vi "STARLYTE.vi"() -> ()   [LabVIEW 2013]
doc: "# STARLYTE AI ENERGY SYSTEM\n# SUBMITTED FOR 2017 NASA INTERNATIONAL SPACE APPS CHALLENGE\n# PROJECT: STARLYTE\n# AUTHORS: ANDREW DENIO, KEVIN JOHNSON\n# DATE: 5/5/2017\n\n\nThis VI demonstrates how to use .Net Speech Recognition to control an application by Voice"
panel:
  out "Battery Storage (%)":dbl(slide) scale=0.0..100.0
  out "TIME":string
  out "Previous 7 Days":T1
  out "12 Day Forecast":T2
  out "Temperature (F)":dbl
  out "Sky Efficiency (%)":dbl
  out "Clearsky GHI (W/m2)":dbl
  in  "offsetHour":i32=-5
  in  "stop":bool
  out "current time":string
  out "current Temperature (deg C)":dbl format="%#_8g"
  out "Solar Radiation-GHI (W/m2)":dbl
  out "Instantaneous Power from the Solar Array":dbl
  out "Dew Point (c)":dbl format="%#_9g"
  out "Pressure (mbar)":dbl format="%#_7g"
  out "Relative Humidity (%)":dbl format="%#_8g"
  out "Precipitable Water (mm)":dbl format="%#_8g"
  out "Wind Direction (degree)":dbl format="%#_7g"
  out "Wind Speed (m/s)":dbl format="%#_9g"
  out "Solar Zenith Angle (degree)":dbl format="%#_7g"
  out "error out 2":errorcluster
  in  "Error in":errorcluster
  out "error out":errorcluster
  out "SpeechLib.ISpeechVoice 2":refnum<k7>
  in  "SpeechLib.ISpeechVoice":refnum<k7>
  out "Score":dbl
  in  "Phrases":i32(listbox)
  in  "Exit":bool
  out "Command":string
  # "HI-SEAS Artificial Intelligence Energy System"
  # "Start Microsoft Speech Engine \nBefore Running this App"
  # "Data for simulation provided by:"
  # "Daily Past Data       -7               -6              -5              -4              -3               -2              -1"
  # "Daily Future Data +1               +2              +3             +4             +5              +6              +7              +8             +9           +10            +11           +12"
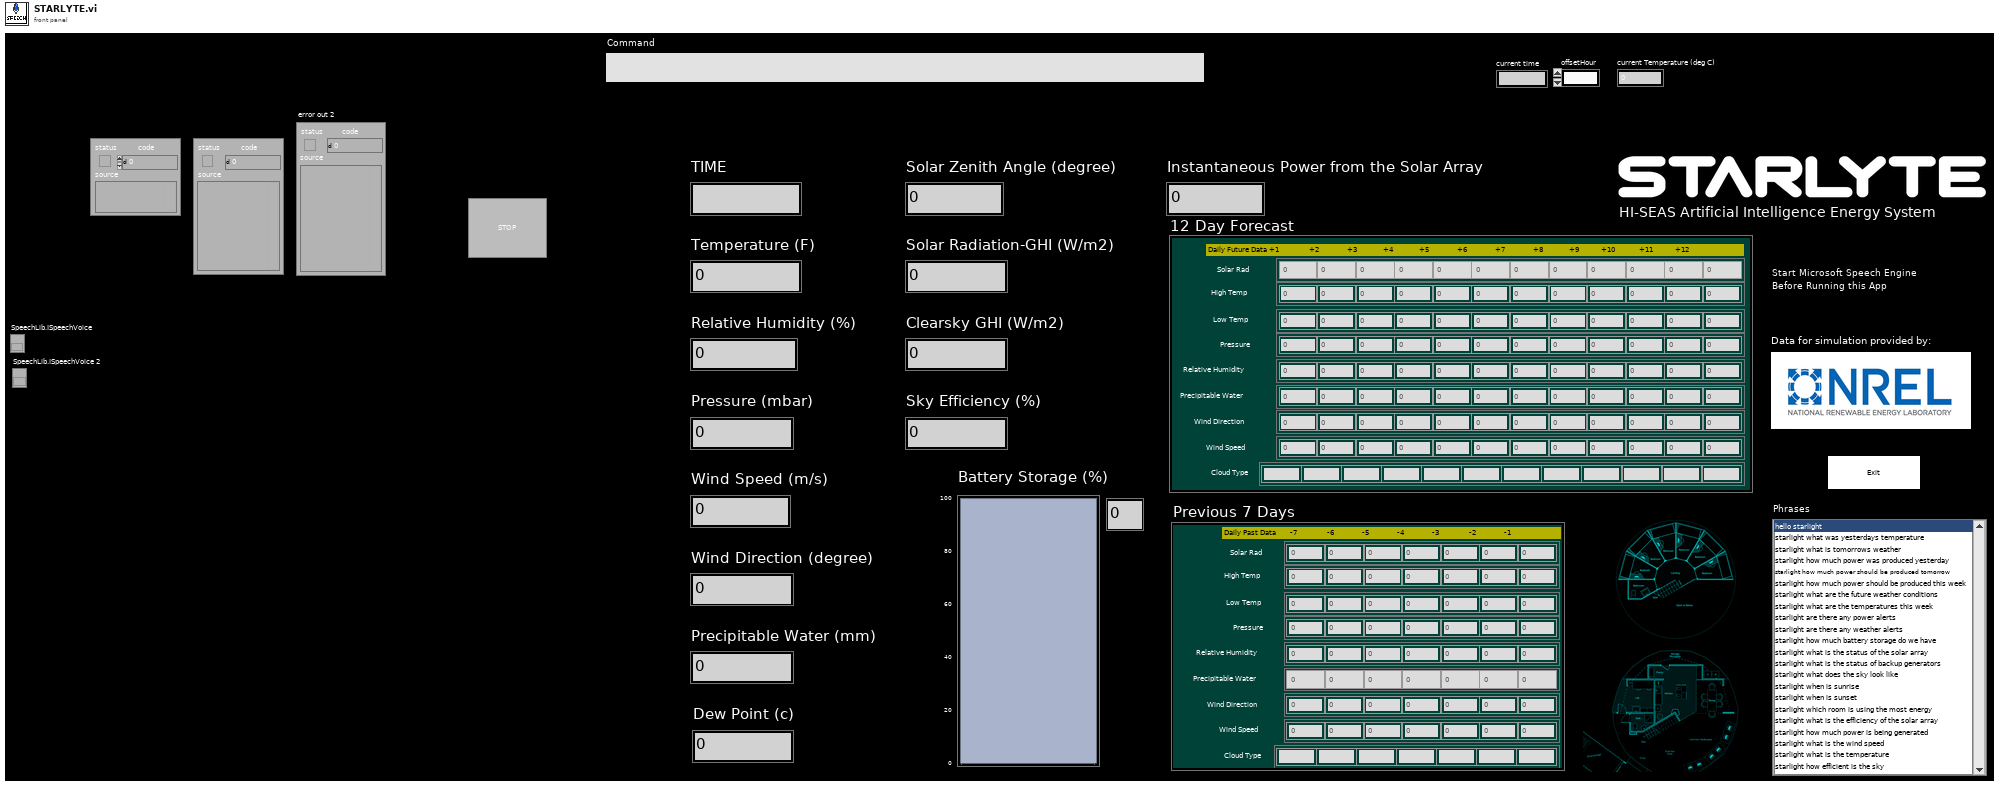
[diagram p1: front panel]
types:
  T1 = cluster{"Wind Speed":dbl[], "Wind Direction":dbl[], "Precipitable Water":dbl[], "Relative Humidity":dbl[], "Pressure":dbl[], "Low Temp":dbl[], "High Temp":dbl[], "Solar Rad":dbl[], "Cloud Type":string[]}
  T2 = cluster{"Solar Rad":dbl[], "High Temp":dbl[], "Low Temp":dbl[], "Pressure":dbl[], "Relative Humidity":dbl[], "Precipitable Water":dbl[], "Wind Direction":dbl[], "Wind Speed":dbl[], "Cloud Type":string[]}
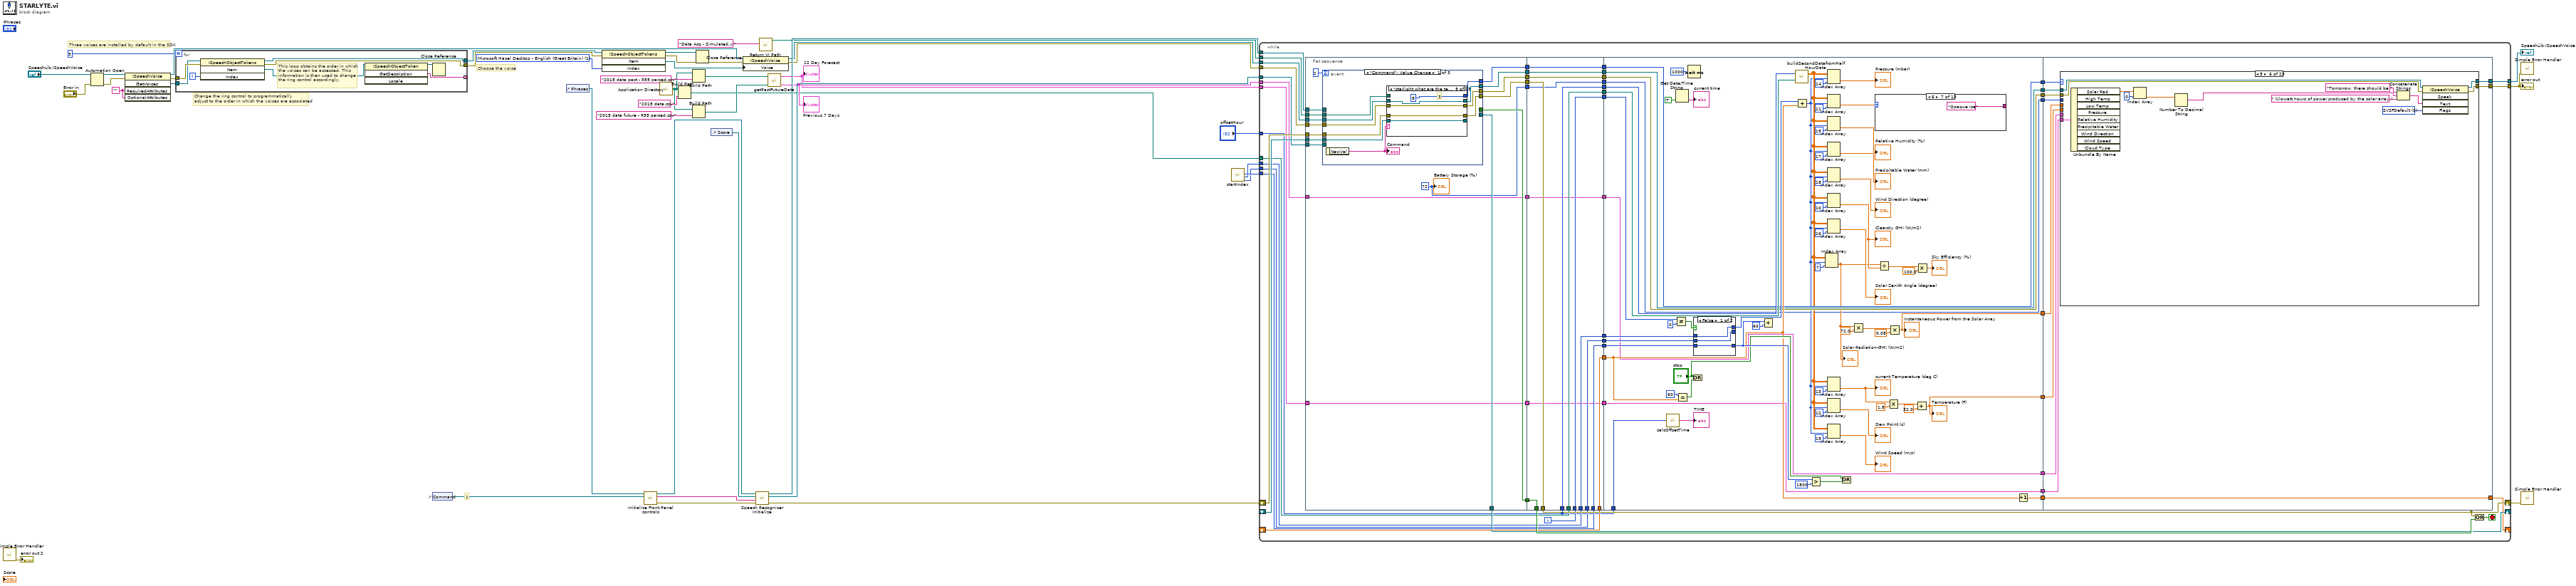
[diagram p0: block diagram]
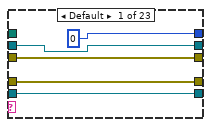
[diagram p2: hidden frame]
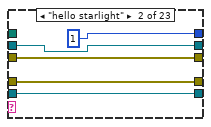
[diagram p3: hidden frame]
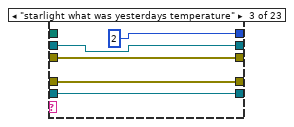
[diagram p4: hidden frame]
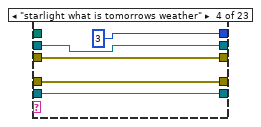
[diagram p5: hidden frame]
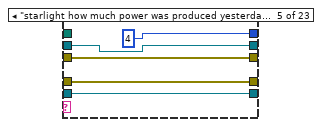
[diagram p6: hidden frame]
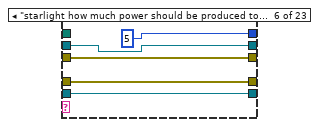
[diagram p7: hidden frame]
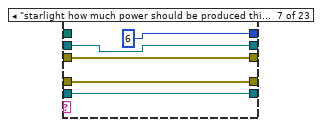
[diagram p8: hidden frame]
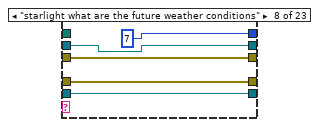
[diagram p9: hidden frame]
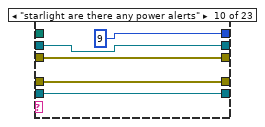
[diagram p10: hidden frame]
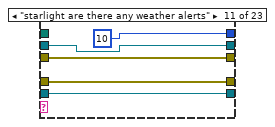
[diagram p11: hidden frame]
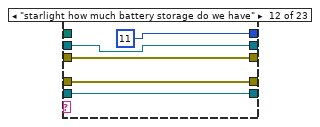
[diagram p12: hidden frame]
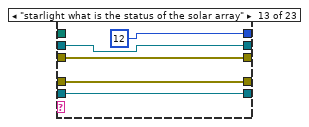
[diagram p13: hidden frame]
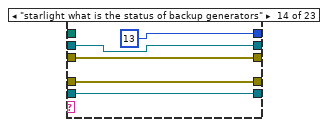
[diagram p14: hidden frame]
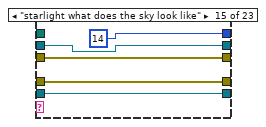
[diagram p15: hidden frame]
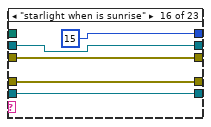
[diagram p16: hidden frame]
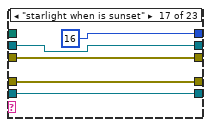
[diagram p17: hidden frame]
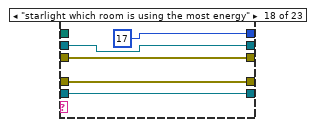
[diagram p18: hidden frame]
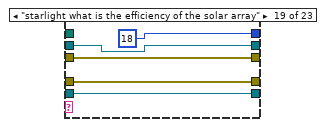
[diagram p19: hidden frame]
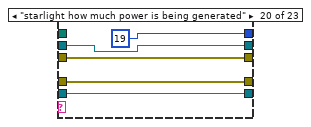
[diagram p20: hidden frame]
diagram:
  w31 = 1 items=["Microsoft David Desktop - English (United States)", "Microsoft Hazel Desktop - English (Great Britain)", "Microsoft Zira Desktop - English (United States)"] ("Choose the voice")
  w29 = ""
  # "Choose the voice"
  # "Three voices are installed by default in the SDK"
  # "Change the ring control to programmatically \nadjust to the order in which the voices are associated"
  # "1"
  n1 = call <vilib>:"Simple Error Handler.vi"() -> ("error out"=→"error out 2":errorcluster)  [unwired: 3 in, 6 out]
  n2 = Automation Open(error in (no error)="Error in", Automation Refnum="SpeechLib.ISpeechVoice") -> (Automation Refnum=w33:refnum<k7>, error out=w28:errorcluster)  [unwired: 2 in]
  n3 = invoke class="ISpeechVoice" method="GetVoices"(reference=w33, error in=w28, "RequiredAttributes"=w29, "OptionalAttributes"=w29) -> (reference out=w32:refnum<k7>, error out=w27:errorcluster, "GetVoices"=w26:refnum<k7>)  [unwired: 1 in, 2 out]
  n4 = for {
    N: 3 -> [_]
    tunnel: [w53] -> w21
    tunnel: w27 -> [w50]
    tunnel: w26 -> [w49]
    tunnel: [w48] -> w24
    tunnel: [w47] -> _ mode=indexing
    i -> [w52]
    # "This loop obtains the order in which\nthe voices can be accessed. This \ninformation is then used to change\nthe ring control accordingly."
    n5 = invoke class="ISpeechObjectTokens" method="Item"(reference=w49, error in=w50, "Index"=w52) -> (reference out=w48:refnum<k7>, error out=w53:errorcluster, "Item"=w54:refnum<k7>)  [unwired: 1 in, 1 out]
    n6 = invoke class="ISpeechObjectToken" method="GetDescription"(reference=w54) -> (reference out=w51:refnum<k7>, "GetDescription"=w47:string)  [unwired: 3 in, 2 out]
    n7 = Close Reference(reference=w51) -> ()  [unwired: 1 in, 1 out]
  }
  n8 = control-ref of="Command"() -> (w40:refnum<vi>)
  n9 = control-ref of="Phrases"() -> (w37:refnum<vi>)
  n10 = invoke class="ISpeechObjectTokens" method="Item"(reference=w24, error in=w21, "Index"=w31) -> (reference out=w23:refnum<k7>, error out=w20:errorcluster, "Item"=w30:refnum<k7>)  [unwired: 1 in, 1 out]
  n11 = call "Initialize Front Panel controls.vi"("Command"=w40, "ListBox in"=w37) -> ("error out"=w38:errorcluster, "Item Names"=w43:string[], "String out"=w41:refnum<vi>)  [unwired: 7 in]
  n12 = call <vilib>:"Application Directory.vi"() -> ("Application Directory"=w4:path)
  n13 = Build Path(base path=w4, name or relative path="2015 data.csv") -> (appended path=w1:path)
  n14 = Build Path(base path=w4, name or relative path="2015 data past - R55 parsed.csv") -> (appended path=w6:path)
  n15 = Build Path(base path=w4, name or relative path="2015 data future - R55 parsed.csv") -> (appended path=w5:path)
  n16 = Close Reference(reference=w23, error in (no error)=w20) -> (error out=w19:errorcluster)
  n17 = control-ref of="Score"() -> (w39:refnum<vi>)
  n18 = property class="ISpeechVoice"(reference=w32, error in=w19, "Voice"=w30) -> (reference out=w18:refnum<k7>, error out=w17:errorcluster)
  n19 = call "Speech Recognizer Initialize.vi"("Error In"=w38, "String[] phrases"=w43, "Score"=w39, "Text"=w41) -> ("error out"=w46:errorcluster, "Event Callback"=w45:refnum<k27>, "reference"=w44:refnum<k24>)  [unwired: 5 out]
  n20 = call "Return VI Path.vi"("name or relative path"="Data Acq - Simulated.vi") -> ("appended path"=w42:path)  [unwired: 10 in]
  n21 = call "getPastFutureData.vi"("2015 data future - R55 parsed.csv"=w5, "2015 data past - R55 parsed.csv"=w6) -> ("Data Past Cluster"=w3:T1, "Data Future Cluster"=w2:T2)  [unwired: 2 in]
  "12 Day Forecast" <- w2
  "Previous 7 Days" <- w3
  n22 = call "startIndex.vi"() -> ("Second"=w10:i32, "startIndex"=w11:i32, "minuteTOsecondStartIndex"=w12:i32)  [unwired: 4 in, 1 out]
  n23 = while {
    shift-right: [w99] -> w35
    shift-left: w46 -> [w107]
    tunnel: w45 -> [w105]
    tunnel: w44 -> [w104]
    tunnel: w42 -> [w103]
    shift-right: [w102] -> _
    shift-left: _ -> [w101]
    tunnel: w18 -> [w98]
    tunnel: w17 -> [w97]
    tunnel: [w72] -> w16
    tunnel: [w73] -> w15
    tunnel: "offsetHour" -> [w60]
    tunnel: w1 -> [w91]
    tunnel: w12 -> [w88]
    tunnel: w11 -> [w86]
    tunnel: w10 -> [w84]
    shift-right: [w81] -> _
    shift-left: _ -> [w79]
    tunnel: w3 -> [w68]
    tunnel: w2 -> [w61]
    i -> [w82]
    stop <- w100 stop-if-true
    n24 = flat-sequence {
      tunnel: w107 -> [w124]
      tunnel: w105 -> [w122]
      tunnel: w104 -> [w121]
      tunnel: w103 -> [w120]
      tunnel: [w113] -> w102
      tunnel: w101 -> [w119]
      tunnel: w98 -> [w117]
      tunnel: w97 -> [w116]
      tunnel: [w123] -> w96
      tunnel: [w118] -> w95
      tunnel: [w115] -> w94
      tunnel: [w114] -> w93
      tunnel: [w111] -> w69
      tunnel: w68 -> [w110]
      tunnel: [w110] -> w67
      tunnel: [w109] -> w62
      tunnel: w61 -> [w109]
      tunnel: [w108] -> w57
      tunnel: [w268] -> w99
      tunnel: [w269] -> w106
      tunnel: w96 -> [w269]
      tunnel: w95 -> [w268]
      tunnel: w94 -> [w259]
      tunnel: w93 -> [w260]
      tunnel: [w267] -> w92
      tunnel: w60 -> [w267]
      tunnel: w91 -> [w266]
      tunnel: [w266] -> w90
      tunnel: [w265] -> w89
      tunnel: w88 -> [w265]
      tunnel: [w264] -> w87
      tunnel: w86 -> [w264]
      tunnel: [w263] -> w85
      tunnel: w84 -> [w263]
      tunnel: [w262] -> w83
      tunnel: w82 -> [w262]
      tunnel: [w261] -> w80
      tunnel: w79 -> [w261]
      tunnel: [w260] -> w76
      tunnel: [w259] -> w74
      tunnel: [w258] -> w70
      tunnel: w69 -> [w258]
      tunnel: w67 -> [w257]
      tunnel: [w257] -> w65
      tunnel: [w256] -> w63
      tunnel: w62 -> [w256]
      tunnel: [w255] -> w58
      tunnel: w57 -> [w255]
      tunnel: w92 -> [w329]
      tunnel: w90 -> [w328]
      tunnel: w89 -> [w327]
      tunnel: w87 -> [w326]
      tunnel: w85 -> [w325]
      tunnel: w83 -> [w324]
      tunnel: w80 -> [w295]
      tunnel: [w319] -> w78
      tunnel: [w294] -> w77
      tunnel: w76 -> [w294]
      tunnel: [w293] -> w75
      tunnel: w74 -> [w293]
      tunnel: [w291] -> w71
      tunnel: w70 -> [w291]
      tunnel: [w276] -> w66
      tunnel: w65 -> [w276]
      tunnel: [w275] -> w64
      tunnel: w63 -> [w275]
      tunnel: w60 -> [w273]
      tunnel: [w272] -> w59
      tunnel: w58 -> [w272]
      tunnel: [w271] -> w56
      tunnel: [w270] -> w55
      tunnel: [w361] -> w81
      tunnel: w78 -> [w361]
      tunnel: w77 -> [w360]
      tunnel: w75 -> [w359]
      tunnel: [w358] -> w73
      tunnel: [w357] -> w72
      tunnel: w71 -> [w356]
      tunnel: w66 -> [w355]
      tunnel: w64 -> [w354]
      tunnel: w59 -> [w353]
      tunnel: w56 -> [w352]
      tunnel: w55 -> [w351]
      frame #0 {
        w108 = 72
        n25 = event shown="[0] \"Command\": Value Change" {
          selector: _ -> [_ _ _]
          dyn-events: _ -> [_ _ _]
          timeout: 2 -> [_ _ _]
          tunnel: w124 -> [w134 _ w251]
          tunnel: [_ _ "Exit"] -> w123
          tunnel: [w133 _ w251] -> w118
          tunnel: w122 -> [_ _ w253]
          tunnel: w121 -> [_ _ w252]
          tunnel: w120 -> [w131 _ _]
          tunnel: w119 -> [w130 _ _]
          tunnel: w117 -> [w129 _ _]
          tunnel: w116 -> [w128 _ _]
          tunnel: [w127 _ _] -> w115
          tunnel: [w126 _ _] -> w114
          tunnel: [_ _ refnum<vi> refnum ("vi reference")] -> w113
          tunnel: [w125 _ _] -> w111
          event "Command": Value Change {
            # "3"
            n26 = event-data() -> ("NewVal"=w132:string)  [unwired: 1 out]
            "Command" <- w132
            n27 = case shown="\"starlight what are the temperatures this week\"" w132 {
              tunnel: w134 -> [w139 w144 w149 w154 w159 w164 w169 w174 w179 w184 w189 w194 w199 w204 w209 w214 w219 w224 w229 w234 w239 w244 w249]
              tunnel: [w139 w144 w149 w154 w159 w164 w169 w174 w179 w184 w189 w194 w199 w204 w209 w214 w219 w224 w229 w234 w239 w244 w249] -> w133
              tunnel: w131 -> [_ _ _ _ _ _ _ _ _ _ _ _ _ _ _ _ _ _ _ _ _ _ _]
              tunnel: [w138 w143 w148 w153 w158 w163 w168 w173 w178 w183 w188 w193 w198 w203 w208 w213 w218 w223 w228 w233 w238 w243 w248] -> _
              tunnel: w130 -> [w138 w143 w148 w153 w158 w163 w168 w173 w178 w183 w188 w193 w198 w203 w208 w213 w218 w223 w228 w233 w238 w243 w248]
              tunnel: w129 -> [w137 w142 w147 w152 w157 w162 w167 w172 w177 w182 w187 w192 w197 w202 w207 w212 w217 w222 w227 w232 w237 w242 w247]
              tunnel: w128 -> [w136 w141 w146 w151 w156 w161 w166 w171 w176 w181 w186 w191 w196 w201 w206 w211 w216 w221 w226 w231 w236 w241 w246]
              tunnel: [w136 w141 w146 w151 w156 w161 w166 w171 w176 w181 w186 w191 w196 w201 w206 w211 w216 w221 w226 w231 w236 w241 w246] -> w127
              tunnel: [w137 w142 w147 w152 w157 w162 w167 w172 w177 w182 w187 w192 w197 w202 w207 w212 w217 w222 w227 w232 w237 w242 w247] -> w126
              tunnel: [0 1 2 3 4 5 6 7 8 9 10 11 12 13 14 15 16 17 18 19 20 21 22] -> w125
              frame Default {
              }
              frame "hello starlight" {
              }
              frame "starlight what was yesterdays temperature" {
              }
              frame "starlight what is tomorrows weather" {
              }
              frame "starlight how much power was produced yesterday" {
              }
              frame "starlight how much power should be produced tomorrow" {
              }
              frame "starlight how much power should be produced this week" {
              }
              frame "starlight what are the future weather conditions" {
              }
              frame "starlight what are the temperatures this week" {
              }
              frame "starlight are there any power alerts" {
              }
              frame "starlight are there any weather alerts" {
              }
              frame "starlight how much battery storage do we have" {
              }
              frame "starlight what is the status of the solar array" {
              }
              frame "starlight what is the status of backup generators" {
              }
              frame "starlight what does the sky look like" {
              }
              frame "starlight when is sunrise" {
              }
              frame "starlight when is sunset" {
              }
              frame "starlight which room is using the most energy" {
              }
              frame "starlight what is the efficiency of the solar array" {
              }
              frame "starlight how much power is being generated" {
              }
              frame "starlight what is the wind speed" {
              }
              frame "starlight what is the temperature" {
              }
              frame "starlight how efficient is the sky" {
              }
            }
          }
          event Timeout {
            n28 = event-data() -> ()  [unwired: 2 out]
          }
          event "Exit": Value Change {
            # "4"
            n29 = event-data() -> ()  [unwired: 2 out]
            n30 = Unregister For Events(event registration refnum=w253) -> ()  [unwired: 1 in, 1 out]
            n31 = Close Reference(reference=w252) -> ()  [unwired: 1 in, 1 out]
          }
        }
        "Battery Storage (%)" <- w108
      }
      frame #1 {
      }
      frame #2 {
        n32 = call "calcOffsetTime.vi"("Hour Offset"=w273) -> ("currentTimeOffset"=→"TIME":string)  [unwired: 4 in]
        n33 = Not Equal?(x=w324, y=0) -> (x != y?=w331:bool)
        n34 = Get Date/Time String(want seconds? (F)=TRUE) -> (time string=→"current time":string)  [unwired: 2 in, 1 out]
        n35 = Equal?(x=60, y=w295) -> (x = y?=w314:bool)
        n36 = Wait (ms)(milliseconds to wait=u32 1000) -> ()  [unwired: 1 out]
        n37 = Or(x="stop", y=w314) -> ()  [unwired: 1 out]
        n38 = case shown="False" w331 {
          tunnel: w325 -> [w349 _]
          tunnel: [w349 w350] -> _
          tunnel: w327 -> [w348 _]
          tunnel: [w348 w350] -> w332
          tunnel: [w347 w350] -> w333
          tunnel: w326 -> [w347 _]
          frame False {
          }
          frame True {
            w350 = 0 ("x")
          }
        }
        n39 = Add(x=w332, y=60 ("x")) -> ()  [unwired: 1 out]
        n40 = call "buildSecondDatafromHalfHourData.vi"("2015 data.csv"=w328, "offsetHour"=w329) -> ("Array"=w284:dbl[][])  [unwired: 1 in]
        n41 = Add(x=w333, y=w295) -> (x+y=w283:i32)
        n42 = Greater?(x=w332, y=1800 ("x")) -> (0:w323:bool)
        n43 = Index Array(array=w284, index (row)=w283, index (col)=7 ("disabled index (col)")) -> (element=w288:dbl)
        "Solar Radiation-GHI (W/m2)" <- w288
        n44 = Index Array(array=w284, index (row)=w283, index (col)=14 ("disabled index (col)")) -> (element=→"Pressure (mbar)":dbl)
        n45 = Index Array(array=w284, index (row)=w283, index (col)=11 ("disabled index (col)")) -> (element=w281:dbl)
        n46 = Index Array(array=w284, index (row)=w283, index (col)=15 ("disabled index (col)")) -> (element=→"Relative Humidity (%)":dbl)
        n47 = Index Array(array=w284, index (row)=w283, index (col)=17 ("disabled index (col)")) -> (element=→"Precipitable Water (mm)":dbl)
        n48 = Index Array(array=w284, index (row)=w283, index (col)=18 ("disabled index (col)")) -> (element=→"Wind Direction (degree)":dbl)
        n49 = Index Array(array=w284, index (row)=w283, index (col)=10 ("disabled index (col)")) -> (element=w289:dbl)
        "Clearsky GHI (W/m2)" <- w289
        n50 = Index Array(array=w284, index (row)=w283, index (col)=16 ("disabled index (col)")) -> (element=→"Solar Zenith Angle (degree)":dbl)
        n51 = Index Array(array=w284, index (row)=w283, index (col)=13 ("disabled index (col)")) -> (element=w278:dbl)
        "current Temperature (deg C)" <- w278
        n52 = Index Array(array=w284, index (row)=w283, index (col)=12 ("disabled index (col)")) -> (element=→"Dew Point (c)":dbl)
        n53 = Index Array(array=w284, index (row)=w283, index (col)=19 ("disabled index (col)")) -> (element=→"Wind Speed (m/s)":dbl)
        n54 = Or(x="stop", y=w323) -> ()  [unwired: 1 out]
        n55 = Multiply(x=w288, y=72.0) -> (x*y=w303:dbl)
        n56 = case shown="6" w281 {
          tunnel: ["Clear" "Probably Clear" "Fog" "Water" "Super-Cooled Water" "Mixed" "Opaque Ice" "Cirrus" "Overlapping" "Overshooting" "Unknown" "Dust" "Smoke"] -> _
          frame 0 {
          }
          frame 1 {
          }
          frame 2 {
          }
          frame 3 {
          }
          frame 4 {
          }
          frame 5 {
          }
          frame 6 {
          }
          frame 7 {
          }
          frame 8 {
          }
          frame 9 {
          }
          frame 10, Default {
          }
          frame 11 {
          }
          frame 12 {
          }
        }
        n57 = Divide(x=w288, y=w289) -> (x/y=w287:dbl)
        n58 = Multiply(x=w278, y=1.8) -> (x*y=w280:dbl)
        n59 = Multiply(x=w303, y=0.08) -> (x*y=w271:dbl)
        "Instantaneous Power from the Solar Array" <- w271
        n60 = Add(x=w280, y=32.0) -> (x+y=w270:dbl)
        "Temperature (F)" <- w270
        n61 = Multiply(x=w287, y=100.0) -> (x*y=→"Sky Efficiency (%)":dbl)
        n62 = Increment(x=w295) -> (x+1=w319:dbl)
      }
      frame #3 {
        n63 = case shown="5" w356 {
          tunnel: w360 -> [w362 w368 w394 w442 w455 w468 w474 w480 w486 w492 w498 w508 w514 w520 w526 w532 w538 w544 w550 w560 w566 w576 w582]
          tunnel: w359 -> [w363 w367 w393 w441 w454 w467 w473 w479 w485 w491 w497 w507 w513 w519 w525 w531 w537 w543 w549 w559 w565 w575 w581]
          tunnel: [w362 w366 w392 w440 w453 w466 w472 w478 w484 w490 w496 w506 w512 w518 w524 w530 w536 w542 w548 w558 w564 w574 w580] -> w358
          tunnel: [w363 w365 w391 w439 w452 w465 w471 w477 w483 w489 w495 w505 w511 w517 w523 w529 w535 w541 w547 w557 w563 w573 w579] -> w357
          tunnel: w355 -> [_ _ w390 _ w451 _ _ _ _ _ _ _ _ _ _ _ _ _ _ _ _ _ _]
          tunnel: w354 -> [_ _ _ w438 _ w464 _ _ _ _ _ _ _ _ _ _ _ _ _ _ _ _ _]
          tunnel: w353 -> [_ _ _ _ _ _ _ _ _ _ _ w503 _ _ _ _ _ _ _ _ _ _ _]
          tunnel: w352 -> [_ _ _ _ _ _ _ _ _ _ _ _ _ _ _ _ _ _ _ w556 _ _ _]
          tunnel: w351 -> [_ _ _ _ _ _ _ _ _ _ _ _ _ _ _ _ _ _ _ _ _ w569 _]
          frame 0, Default {
          }
          frame 1 {
            w369 = 0 items=["SVSFDefault"=0, "SVSFlagsAsync"=1, "SVSFPurgeBeforeSpeak"=2, "SVSFIsFilename"=4, "SVSFIsXML"=8, "SVSFIsNotXML"=16, "SVSFPersistXML"=32, "SVSFNLPSpeakPunc, SVSFNLPMask"=64, "SVSFVoiceMask"=127, "SVSFUnusedFlags"=-128] ("Flags")
            n64 = invoke class="ISpeechVoice" method="Speak"(reference=w368, error in=w367, "Text"="Hello crew mate Denio", "Flags"=w369) -> (reference out=w366:refnum<k7>, error out=w365:errorcluster)  [unwired: 1 in, 3 out]
          }
          frame 2 {
            w395 = 0 items=["SVSFDefault"=0, "SVSFlagsAsync"=1, "SVSFPurgeBeforeSpeak"=2, "SVSFIsFilename"=4, "SVSFIsXML"=8, "SVSFIsNotXML"=16, "SVSFPersistXML"=32, "SVSFNLPSpeakPunc, SVSFNLPMask"=64, "SVSFVoiceMask"=127, "SVSFUnusedFlags"=-128] ("Flags")
            n65 = Unbundle By Name(w390) -> ("Low Temp"=w389:dbl[], "High Temp"=w386:dbl[])  [unwired: 7 out]
            n66 = Index Array(array=w386, index=6) -> (element=w375:dbl)
            n67 = Index Array(array=w389, index=6) -> (element=w381:dbl)
            n68 = Multiply(x=w375, y=1.8) -> (x*y=w378:dbl)
            n69 = Multiply(x=w381, y=1.8) -> (x*y=w382:dbl)
            n70 = Add(x=w378, y=32.0) -> (x+y=w379:dbl)
            n71 = Add(x=w382, y=32.0) -> (x+y=w380:dbl)
            n72 = Number To Decimal String(number=w379) -> (decimal integer string=w374:string)  [unwired: 1 in]
            n73 = Number To Decimal String(number=w380) -> (decimal integer string=w372:string)  [unwired: 1 in]
            n74 = Concatenate Strings("Yesterday, the high temperature was " ("string"), w374, " degrees farenheit and the low temperature was " ("string"), w372, " degrees farenheit" ("string")) -> (w370:string)
            n75 = invoke class="ISpeechVoice" method="Speak"(reference=w394, error in=w393, "Text"=w370, "Flags"=w395) -> (reference out=w392:refnum<k7>, error out=w391:errorcluster)  [unwired: 1 in, 3 out]
          }
          frame 3 {
            w443 = 0 items=["SVSFDefault"=0, "SVSFlagsAsync"=1, "SVSFPurgeBeforeSpeak"=2, "SVSFIsFilename"=4, "SVSFIsXML"=8, "SVSFIsNotXML"=16, "SVSFPersistXML"=32, "SVSFNLPSpeakPunc, SVSFNLPMask"=64, "SVSFVoiceMask"=127, "SVSFUnusedFlags"=-128] ("Flags")
            n76 = Unbundle By Name(w438) -> ("Solar Rad"=w423:dbl[], "High Temp"=w431:dbl[], "Low Temp"=w424:dbl[], "Pressure"=w418:dbl[], "Relative Humidity"=w414:dbl[], "Precipitable Water"=w410:dbl[], "Wind Direction"=w406:dbl[], "Wind Speed"=w413:dbl[])  [unwired: 1 out]
            n77 = Index Array(array=w431, index=0) -> (element=w436:dbl)
            n78 = Index Array(array=w424, index=0) -> (element=w426:dbl)
            n79 = Index Array(array=w423, index=0) -> (element=w421:dbl)
            n80 = Index Array(array=w418, index=0) -> (element=w419:dbl)
            n81 = Index Array(array=w414, index=0) -> (element=w412:dbl)
            n82 = Index Array(array=w410, index=0) -> (element=w409:dbl)
            n83 = Index Array(array=w406, index=0) -> (element=w408:dbl)
            n84 = Index Array(array=w413, index=0) -> (element=w411:dbl)
            n85 = Number To Decimal String(number=w421) -> ()  [unwired: 1 in, 1 out]
            n86 = Number To Decimal String(number=w419) -> ()  [unwired: 1 in, 1 out]
            n87 = Number To Decimal String(number=w409) -> ()  [unwired: 1 in, 1 out]
            n88 = Number To Decimal String(number=w408) -> ()  [unwired: 1 in, 1 out]
            n89 = Number To Decimal String(number=w412) -> (decimal integer string=w399:string)  [unwired: 1 in]
            n90 = Number To Decimal String(number=w411) -> (decimal integer string=w396:string)  [unwired: 1 in]
            n91 = Multiply(x=w436, y=1.8) -> (x*y=w435:dbl)
            n92 = Multiply(x=w426, y=1.8) -> (x*y=w427:dbl)
            n93 = Add(x=w435, y=32.0) -> (x+y=w437:dbl)
            n94 = Add(x=w427, y=32.0) -> (x+y=w425:dbl)
            n95 = Number To Decimal String(number=w437) -> (decimal integer string=w404:string)  [unwired: 1 in]
            n96 = Number To Decimal String(number=w425) -> (decimal integer string=w401:string)  [unwired: 1 in]
            n97 = Concatenate Strings("Tomrrow, the high temperature will be " ("string"), w404, " degrees farenheit, and the low temperature will be " ("string"), w401, " degrees farenheit, The humidity will be " ("string"), w399, " percent, and the wind speed will reach " ("string"), w396, " miles per hour." ("string")) -> (w402:string)
            n98 = invoke class="ISpeechVoice" method="Speak"(reference=w442, error in=w441, "Text"=w402, "Flags"=w443) -> (reference out=w440:refnum<k7>, error out=w439:errorcluster)  [unwired: 1 in, 3 out]
          }
          frame 4 {
            w456 = 0 items=["SVSFDefault"=0, "SVSFlagsAsync"=1, "SVSFPurgeBeforeSpeak"=2, "SVSFIsFilename"=4, "SVSFIsXML"=8, "SVSFIsNotXML"=16, "SVSFPersistXML"=32, "SVSFNLPSpeakPunc, SVSFNLPMask"=64, "SVSFVoiceMask"=127, "SVSFUnusedFlags"=-128] ("Flags")
            n99 = Unbundle By Name(w451) -> ("Solar Rad"=w448:dbl[])  [unwired: 8 out]
            n100 = Index Array(array=w448, index=0) -> (element=w450:dbl)
            n101 = Number To Decimal String(number=w450) -> (decimal integer string=w446:string)  [unwired: 1 in]
            n102 = Concatenate Strings("Yesterday, there were " ("string"), w446, " kilowatt hours produced from the solar array." ("string")) -> (w444:string)
            n103 = invoke class="ISpeechVoice" method="Speak"(reference=w455, error in=w454, "Text"=w444, "Flags"=w456) -> (reference out=w453:refnum<k7>, error out=w452:errorcluster)  [unwired: 1 in, 3 out]
          }
          frame 5 {
            w469 = 0 items=["SVSFDefault"=0, "SVSFlagsAsync"=1, "SVSFPurgeBeforeSpeak"=2, "SVSFIsFilename"=4, "SVSFIsXML"=8, "SVSFIsNotXML"=16, "SVSFPersistXML"=32, "SVSFNLPSpeakPunc, SVSFNLPMask"=64, "SVSFVoiceMask"=127, "SVSFUnusedFlags"=-128] ("Flags")
            n104 = Unbundle By Name(w464) -> ("Solar Rad"=w463:dbl[])  [unwired: 8 out]
            n105 = Index Array(array=w463, index=0) -> (element=w461:dbl)
            n106 = Number To Decimal String(number=w461) -> (decimal integer string=w458:string)  [unwired: 1 in]
            n107 = Concatenate Strings("Tomorrow, there should be " ("string"), w458, " kilowatt hours of power produced by the solar array." ("string")) -> (w460:string)
            n108 = invoke class="ISpeechVoice" method="Speak"(reference=w468, error in=w467, "Text"=w460, "Flags"=w469) -> (reference out=w466:refnum<k7>, error out=w465:errorcluster)  [unwired: 1 in, 3 out]
          }
          frame 6 {
            w475 = 0 items=["SVSFDefault"=0, "SVSFlagsAsync"=1, "SVSFPurgeBeforeSpeak"=2, "SVSFIsFilename"=4, "SVSFIsXML"=8, "SVSFIsNotXML"=16, "SVSFPersistXML"=32, "SVSFNLPSpeakPunc, SVSFNLPMask"=64, "SVSFVoiceMask"=127, "SVSFUnusedFlags"=-128] ("Flags")
            n109 = invoke class="ISpeechVoice" method="Speak"(reference=w474, error in=w473, "Text"=" ", "Flags"=w475) -> (reference out=w472:refnum<k7>, error out=w471:errorcluster)  [unwired: 1 in, 3 out]
          }
          frame 7 {
            w481 = 0 items=["SVSFDefault"=0, "SVSFlagsAsync"=1, "SVSFPurgeBeforeSpeak"=2, "SVSFIsFilename"=4, "SVSFIsXML"=8, "SVSFIsNotXML"=16, "SVSFPersistXML"=32, "SVSFNLPSpeakPunc, SVSFNLPMask"=64, "SVSFVoiceMask"=127, "SVSFUnusedFlags"=-128] ("Flags")
            n110 = invoke class="ISpeechVoice" method="Speak"(reference=w480, error in=w479, "Text"=" ", "Flags"=w481) -> (reference out=w478:refnum<k7>, error out=w477:errorcluster)  [unwired: 1 in, 3 out]
          }
          frame 8 {
            w487 = 0 items=["SVSFDefault"=0, "SVSFlagsAsync"=1, "SVSFPurgeBeforeSpeak"=2, "SVSFIsFilename"=4, "SVSFIsXML"=8, "SVSFIsNotXML"=16, "SVSFPersistXML"=32, "SVSFNLPSpeakPunc, SVSFNLPMask"=64, "SVSFVoiceMask"=127, "SVSFUnusedFlags"=-128] ("Flags")
            n111 = invoke class="ISpeechVoice" method="Speak"(reference=w486, error in=w485, "Text"=" ", "Flags"=w487) -> (reference out=w484:refnum<k7>, error out=w483:errorcluster)  [unwired: 1 in, 3 out]
          }
          frame 9 {
            w493 = 0 items=["SVSFDefault"=0, "SVSFlagsAsync"=1, "SVSFPurgeBeforeSpeak"=2, "SVSFIsFilename"=4, "SVSFIsXML"=8, "SVSFIsNotXML"=16, "SVSFPersistXML"=32, "SVSFNLPSpeakPunc, SVSFNLPMask"=64, "SVSFVoiceMask"=127, "SVSFUnusedFlags"=-128] ("Flags")
            n112 = invoke class="ISpeechVoice" method="Speak"(reference=w492, error in=w491, "Text"="There are no power alerts, Solar array performance is optimal ", "Flags"=w493) -> (reference out=w490:refnum<k7>, error out=w489:errorcluster)  [unwired: 1 in, 3 out]
          }
          frame 10 {
            w499 = 0 items=["SVSFDefault"=0, "SVSFlagsAsync"=1, "SVSFPurgeBeforeSpeak"=2, "SVSFIsFilename"=4, "SVSFIsXML"=8, "SVSFIsNotXML"=16, "SVSFPersistXML"=32, "SVSFNLPSpeakPunc, SVSFNLPMask"=64, "SVSFVoiceMask"=127, "SVSFUnusedFlags"=-128] ("Flags")
            n113 = invoke class="ISpeechVoice" method="Speak"(reference=w498, error in=w497, "Text"="There are no weather alerts at this time. ", "Flags"=w499) -> (reference out=w496:refnum<k7>, error out=w495:errorcluster)  [unwired: 1 in, 3 out]
          }
          frame 11 {
            w509 = 0 items=["SVSFDefault"=0, "SVSFlagsAsync"=1, "SVSFPurgeBeforeSpeak"=2, "SVSFIsFilename"=4, "SVSFIsXML"=8, "SVSFIsNotXML"=16, "SVSFPersistXML"=32, "SVSFNLPSpeakPunc, SVSFNLPMask"=64, "SVSFVoiceMask"=127, "SVSFUnusedFlags"=-128] ("Flags")
            n114 = Number To Decimal String(number=w503) -> (decimal integer string=w502:string)  [unwired: 1 in]
            n115 = Concatenate Strings("The battery storage is currently at " ("string"), w502, " percent" ("string")) -> (w500:string)
            n116 = invoke class="ISpeechVoice" method="Speak"(reference=w508, error in=w507, "Text"=w500, "Flags"=w509) -> (reference out=w506:refnum<k7>, error out=w505:errorcluster)  [unwired: 1 in, 3 out]
          }
          frame 12 {
            w515 = 0 items=["SVSFDefault"=0, "SVSFlagsAsync"=1, "SVSFPurgeBeforeSpeak"=2, "SVSFIsFilename"=4, "SVSFIsXML"=8, "SVSFIsNotXML"=16, "SVSFPersistXML"=32, "SVSFNLPSpeakPunc, SVSFNLPMask"=64, "SVSFVoiceMask"=127, "SVSFUnusedFlags"=-128] ("Flags")
            n117 = invoke class="ISpeechVoice" method="Speak"(reference=w514, error in=w513, "Text"="The solar array is functional, but panel number twenty five is below specifications ", "Flags"=w515) -> (reference out=w512:refnum<k7>, error out=w511:errorcluster)  [unwired: 1 in, 3 out]
          }
          frame 13 {
            w521 = 0 items=["SVSFDefault"=0, "SVSFlagsAsync"=1, "SVSFPurgeBeforeSpeak"=2, "SVSFIsFilename"=4, "SVSFIsXML"=8, "SVSFIsNotXML"=16, "SVSFPersistXML"=32, "SVSFNLPSpeakPunc, SVSFNLPMask"=64, "SVSFVoiceMask"=127, "SVSFUnusedFlags"=-128] ("Flags")
            n118 = invoke class="ISpeechVoice" method="Speak"(reference=w520, error in=w519, "Text"=" ", "Flags"=w521) -> (reference out=w518:refnum<k7>, error out=w517:errorcluster)  [unwired: 1 in, 3 out]
          }
          frame 14 {
            w527 = 0 items=["SVSFDefault"=0, "SVSFlagsAsync"=1, "SVSFPurgeBeforeSpeak"=2, "SVSFIsFilename"=4, "SVSFIsXML"=8, "SVSFIsNotXML"=16, "SVSFPersistXML"=32, "SVSFNLPSpeakPunc, SVSFNLPMask"=64, "SVSFVoiceMask"=127, "SVSFUnusedFlags"=-128] ("Flags")
            n119 = invoke class="ISpeechVoice" method="Speak"(reference=w526, error in=w525, "Text"=" ", "Flags"=w527) -> (reference out=w524:refnum<k7>, error out=w523:errorcluster)  [unwired: 1 in, 3 out]
          }
          frame 15 {
            w533 = 0 items=["SVSFDefault"=0, "SVSFlagsAsync"=1, "SVSFPurgeBeforeSpeak"=2, "SVSFIsFilename"=4, "SVSFIsXML"=8, "SVSFIsNotXML"=16, "SVSFPersistXML"=32, "SVSFNLPSpeakPunc, SVSFNLPMask"=64, "SVSFVoiceMask"=127, "SVSFUnusedFlags"=-128] ("Flags")
            n120 = invoke class="ISpeechVoice" method="Speak"(reference=w532, error in=w531, "Text"="Tomorrow, the sunrise will occur at five fifty two a m ", "Flags"=w533) -> (reference out=w530:refnum<k7>, error out=w529:errorcluster)  [unwired: 1 in, 3 out]
          }
          frame 16 {
            w539 = 0 items=["SVSFDefault"=0, "SVSFlagsAsync"=1, "SVSFPurgeBeforeSpeak"=2, "SVSFIsFilename"=4, "SVSFIsXML"=8, "SVSFIsNotXML"=16, "SVSFPersistXML"=32, "SVSFNLPSpeakPunc, SVSFNLPMask"=64, "SVSFVoiceMask"=127, "SVSFUnusedFlags"=-128] ("Flags")
            n121 = invoke class="ISpeechVoice" method="Speak"(reference=w538, error in=w537, "Text"="Tonight, sunset will occur at six forty three p m ", "Flags"=w539) -> (reference out=w536:refnum<k7>, error out=w535:errorcluster)  [unwired: 1 in, 3 out]
          }
          frame 17 {
            w545 = 0 items=["SVSFDefault"=0, "SVSFlagsAsync"=1, "SVSFPurgeBeforeSpeak"=2, "SVSFIsFilename"=4, "SVSFIsXML"=8, "SVSFIsNotXML"=16, "SVSFPersistXML"=32, "SVSFNLPSpeakPunc, SVSFNLPMask"=64, "SVSFVoiceMask"=127, "SVSFUnusedFlags"=-128] ("Flags")
            n122 = invoke class="ISpeechVoice" method="Speak"(reference=w544, error in=w543, "Text"="The current room using the most energy is the kitchen. ", "Flags"=w545) -> (reference out=w542:refnum<k7>, error out=w541:errorcluster)  [unwired: 1 in, 3 out]
          }
          frame 18 {
            w551 = 0 items=["SVSFDefault"=0, "SVSFlagsAsync"=1, "SVSFPurgeBeforeSpeak"=2, "SVSFIsFilename"=4, "SVSFIsXML"=8, "SVSFIsNotXML"=16, "SVSFPersistXML"=32, "SVSFNLPSpeakPunc, SVSFNLPMask"=64, "SVSFVoiceMask"=127, "SVSFUnusedFlags"=-128] ("Flags")
            n123 = invoke class="ISpeechVoice" method="Speak"(reference=w550, error in=w549, "Text"=" ", "Flags"=w551) -> (reference out=w548:refnum<k7>, error out=w547:errorcluster)  [unwired: 1 in, 3 out]
          }
          frame 19 {
            w561 = 0 items=["SVSFDefault"=0, "SVSFlagsAsync"=1, "SVSFPurgeBeforeSpeak"=2, "SVSFIsFilename"=4, "SVSFIsXML"=8, "SVSFIsNotXML"=16, "SVSFPersistXML"=32, "SVSFNLPSpeakPunc, SVSFNLPMask"=64, "SVSFVoiceMask"=127, "SVSFUnusedFlags"=-128] ("Flags")
            n124 = Number To Decimal String(number=w556) -> (decimal integer string=w554:string)  [unwired: 1 in]
            n125 = Concatenate Strings("Right now, there are " ("string"), w554, " watts being produced by the solar array" ("string")) -> (w552:string)
            n126 = invoke class="ISpeechVoice" method="Speak"(reference=w560, error in=w559, "Text"=w552, "Flags"=w561) -> (reference out=w558:refnum<k7>, error out=w557:errorcluster)  [unwired: 1 in, 3 out]
          }
          frame 20 {
            w567 = 0 items=["SVSFDefault"=0, "SVSFlagsAsync"=1, "SVSFPurgeBeforeSpeak"=2, "SVSFIsFilename"=4, "SVSFIsXML"=8, "SVSFIsNotXML"=16, "SVSFPersistXML"=32, "SVSFNLPSpeakPunc, SVSFNLPMask"=64, "SVSFVoiceMask"=127, "SVSFUnusedFlags"=-128] ("Flags")
            n127 = invoke class="ISpeechVoice" method="Speak"(reference=w566, error in=w565, "Text"=" ", "Flags"=w567) -> (reference out=w564:refnum<k7>, error out=w563:errorcluster)  [unwired: 1 in, 3 out]
          }
          frame 21 {
            w577 = 0 items=["SVSFDefault"=0, "SVSFlagsAsync"=1, "SVSFPurgeBeforeSpeak"=2, "SVSFIsFilename"=4, "SVSFIsXML"=8, "SVSFIsNotXML"=16, "SVSFPersistXML"=32, "SVSFNLPSpeakPunc, SVSFNLPMask"=64, "SVSFVoiceMask"=127, "SVSFUnusedFlags"=-128] ("Flags")
            n128 = Number To Decimal String(number=w569) -> (decimal integer string=w571:string)  [unwired: 1 in]
            n129 = Concatenate Strings("The current temperature is " ("string"), w571, " degrees farenheit." ("string")) -> (w568:string)
            n130 = invoke class="ISpeechVoice" method="Speak"(reference=w576, error in=w575, "Text"=w568, "Flags"=w577) -> (reference out=w574:refnum<k7>, error out=w573:errorcluster)  [unwired: 1 in, 3 out]
          }
          frame 22 {
            w583 = 0 items=["SVSFDefault"=0, "SVSFlagsAsync"=1, "SVSFPurgeBeforeSpeak"=2, "SVSFIsFilename"=4, "SVSFIsXML"=8, "SVSFIsNotXML"=16, "SVSFPersistXML"=32, "SVSFNLPSpeakPunc, SVSFNLPMask"=64, "SVSFVoiceMask"=127, "SVSFUnusedFlags"=-128] ("Flags")
            n131 = invoke class="ISpeechVoice" method="Speak"(reference=w582, error in=w581, "Text"=" ", "Flags"=w583) -> (reference out=w580:refnum<k7>, error out=w579:errorcluster)  [unwired: 1 in, 3 out]
          }
        }
      }
    }
    n132 = Or(x=w99, y=w106) -> (x .or. y?=w100:bool)
  }
  "SpeechLib.ISpeechVoice 2" <- w15
  "error out" <- w16
  n133 = call <vilib>:"Simple Error Handler.vi"("error in (no error)"=w16) -> ()  [unwired: 4 in, 5 out]
  n134 = call <vilib>:"Simple Error Handler.vi"("error in (no error)"=w35) -> ()  [unwired: 4 in, 5 out]
